vi "Thin Etalon Linewidth Sweep Reset.vi"(5 "slide reference":refnum<vi>, 7 "reset":bool, 9 "Right in":i32, 10 "center in":i32, 11 "left in":i32) -> (1 "Right out":i32, 2 "center out":i32, 3 "left out":i32)   [LabVIEW 2013]
panel:
  out "Thin Etalon Position":i32
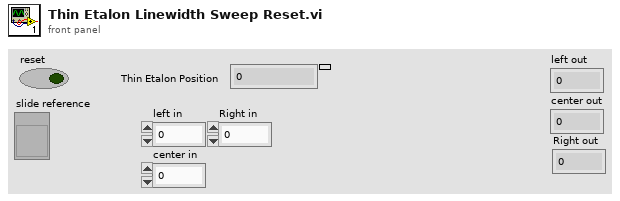
[diagram p1: front panel]
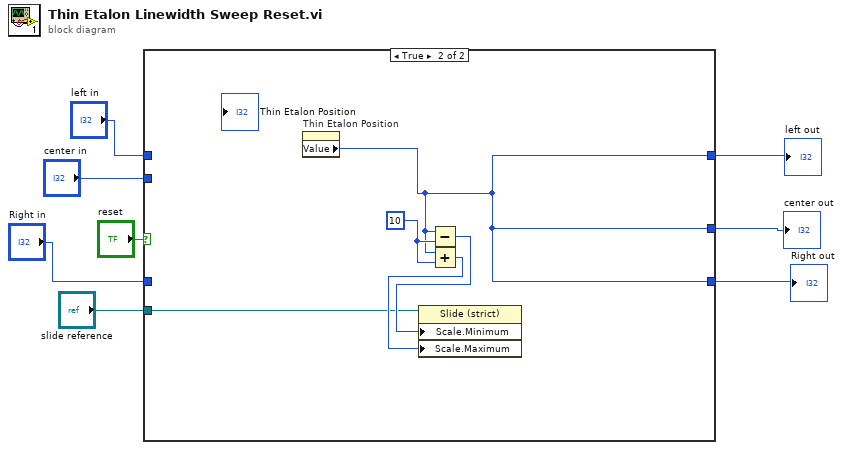
[diagram p0: block diagram]
diagram:
  n1 = case shown="True" "reset" {
    tunnel: "slide reference" -> [_ w13]
    tunnel: [w11 w12] -> w6
    tunnel: [w10 w12] -> w5
    tunnel: [w9 w12] -> w4
    tunnel: "left in" -> [w11 _]
    tunnel: "center in" -> [w10 _]
    tunnel: "Right in" -> [w9 _]
    frame False {
    }
    frame True {
      w15 = 10
      n2 = property on="Thin Etalon Position" class="DigNum (strict)"() -> ("Value"=w12:i32)  [unwired: 2 in, 2 out]
      n3 = Subtract(x=w12, y=w15) -> (x-y=w14:i32)
      n4 = Add(x=w12, y=w15) -> (x+y=w16:i32)
      n5 = property on="Property Node" class="Slide (strict)"(reference=w13, "Scale.Minimum"=w14, "Scale.Maximum"=w16) -> ()  [unwired: 1 in, 2 out]
    }
  }
  "left out" <- w6
  "center out" <- w5
  "Right out" <- w4
